vi "banda.vi"() -> ()   [LabVIEW 2020]
uses:
  Control 4.ctl
  <vilib>/Utility/miscctls.llb/LVPointTypeDef.ctl
panel:
  in  "Speed":u8=1
  out "Indicadores":T1
  in  "Start":bool
  in  "Slide":u8(slide) scale=0.0..100.0
  out "Sensores":T2
  # "41-59"
  # "ON"
  # "OFF"
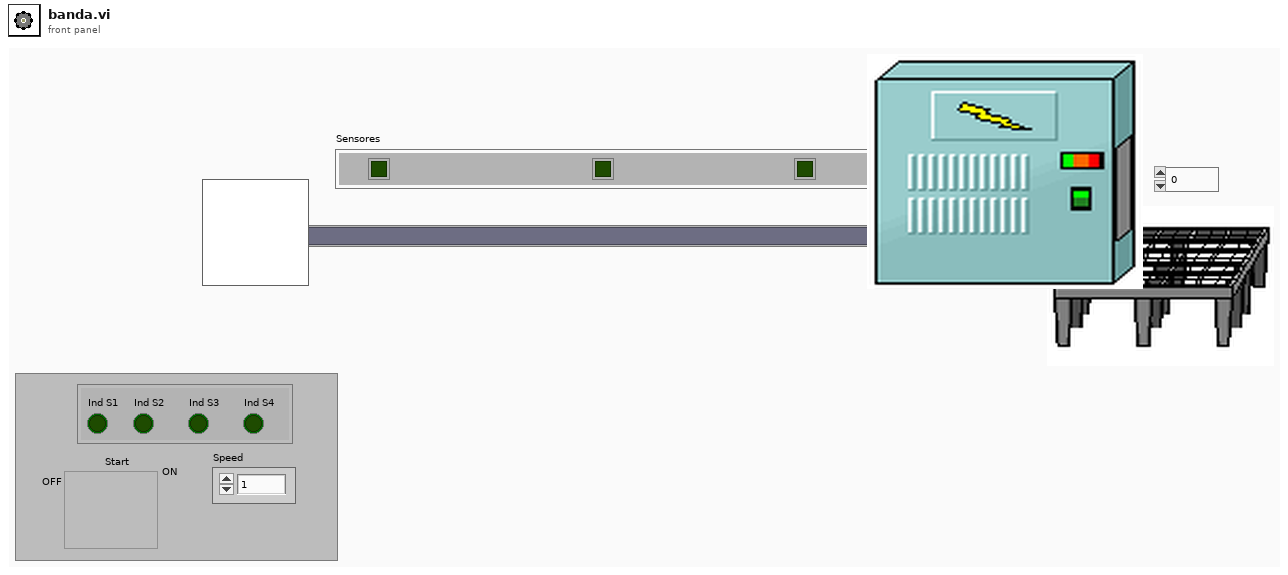
[diagram p1: front panel]
types:
  T1 = cluster{"Ind S1":bool, "Ind S2":bool, "Ind S3":bool, "Ind S4":bool}
  T2 = cluster{"S1":bool, "S2":bool, "S3":bool, "S4":bool}
  T3 = typedef "LVPointTypeDef.ctl" = cluster{"Horizontal":i16, "Vertical":i16}
  T4 = typedef "Control 4.ctl" = enum16{"inicializar", "avanzar", "parar", "verificar"}
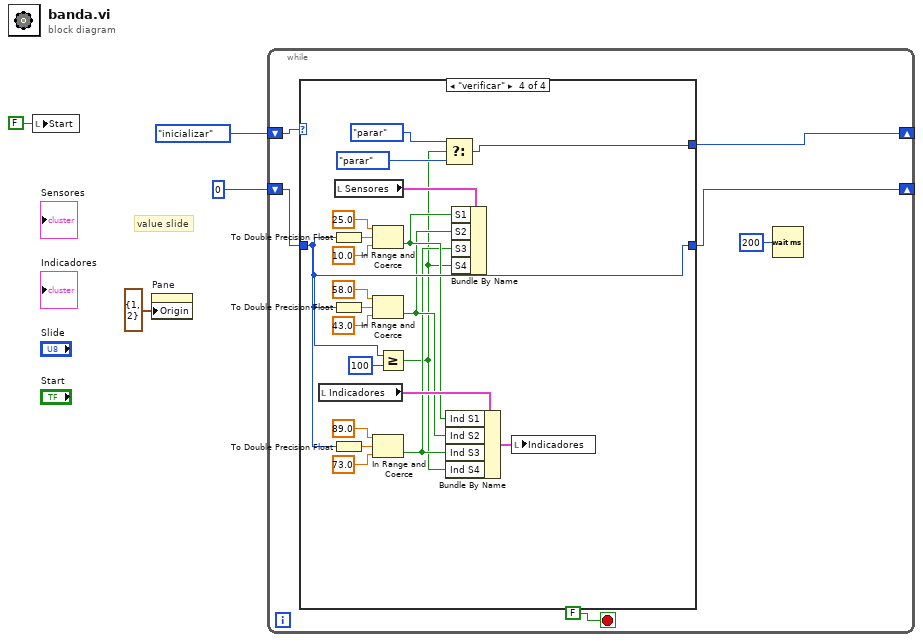
[diagram p0: block diagram]
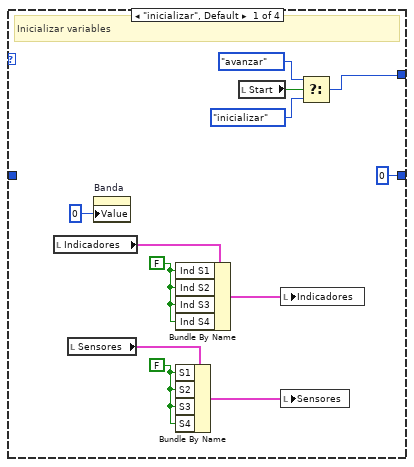
[diagram p2: hidden frame]
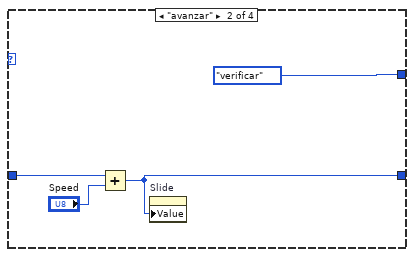
[diagram p3: hidden frame]
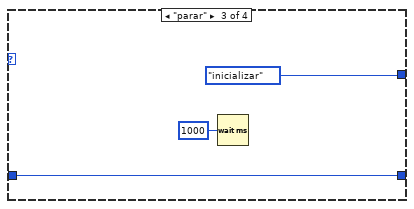
[diagram p4: hidden frame]
diagram:
  # "value slide"
  n1 = local write "Start"(FALSE ("Start")) -> ()
  n2 = property on="Pane" class="Pane"("Origin"=T3 {"Horizontal"=1, "Vertical"=2}) -> ()  [unwired: 2 in, 2 out]
  n3 = while {
    shift-right: [w9] -> _
    shift-left: Control_4."inicializar" -> [w10]
    shift-right: [w7] -> _
    shift-left: u8 0 -> [w8]
    stop <- FALSE stop-if-true
    n4 = case shown="\"verificar\"" w10 {
      tunnel: [w12 Control_4."verificar" Control_4."inicializar" w36] -> w9
      tunnel: w8 -> [_ w26 w29 w39]
      tunnel: [u8 0 w24 w29 w39] -> w7
      frame "inicializar", Default {
        w17 = FALSE ("S1")
        w20 = FALSE ("S1")
        # "Inicializar variables"
        n5 = local read "Indicadores"() -> (w16:T1)
        n6 = local read "Sensores"() -> (w21:T2)
        n7 = property on="Banda" class="Slide (strict)"("Value"=u8 0 ("Slide")) -> ()  [unwired: 2 in, 2 out]
        n8 = Bundle By Name(cluster=w16, "Ind S1"=w17, "Ind S2"=w17, "Ind S3"=w17, "Ind S4"=w17) -> (w18:T1)
        n9 = Bundle By Name(cluster=w21, "S1"=w20, "S2"=w20, "S3"=w20, "S4"=w20) -> (w19:T2)
        n10 = local read "Start"() -> (w15:bool)
        n11 = local write "Indicadores"(w18) -> ()
        n12 = local write "Sensores"(w19) -> ()
        n13 = Select(t=Control_4."avanzar", s=w15, f=Control_4."inicializar") -> (s? t:f=w12:T4)
      }
      frame "avanzar" {
        n14 = Add(x=w26, y="Speed") -> (x+y=w24:u8)
        n15 = property on="Slide" class="Slide (strict)"("Value"=w24) -> ()  [unwired: 2 in, 2 out]
      }
      frame "parar" {
        n16 = Wait (ms)(milliseconds to wait=u32 1000) -> ()  [unwired: 1 out]
      }
      frame "verificar" {
        n17 = local read "Indicadores"() -> (w34:T1)
        n18 = To Double Precision Float(number=w39) -> (double precision float=w48:dbl)
        n19 = To Double Precision Float(number=w39) -> (double precision float=w46:dbl)
        n20 = To Double Precision Float(number=w39) -> (double precision float=w41:dbl)
        n21 = local read "Sensores"() -> (w47:T2)
        n22 = In Range and Coerce(upper limit=25.0 ("lower limit"), x=w48, lower limit=10.0) -> (In Range?=w33:bool)  [unwired: 1 out]
        n23 = In Range and Coerce(upper limit=58.0 ("lower limit"), x=w46, lower limit=43.0) -> (In Range?=w32:bool)  [unwired: 1 out]
        n24 = In Range and Coerce(upper limit=89.0 ("lower limit"), x=w41, lower limit=73.0) -> (In Range?=w31:bool)  [unwired: 1 out]
        n25 = Greater Or Equal?(x=w39, y=u8 100 ("lower limit")) -> (x >= y?=w30:bool)
        n26 = Select(t=Control_4."parar", s=w30, f=Control_4."parar") -> (s? t:f=w36:T4)
        n27 = Bundle By Name(cluster=w34, "Ind S1"=w33, "Ind S2"=w32, "Ind S3"=w31, "Ind S4"=w30) -> (w35:T1)
        n28 = Bundle By Name(cluster=w47, "S1"=w33, "S2"=w32, "S3"=w31, "S4"=w30) -> ()  [unwired: 1 out]
        n29 = local write "Indicadores"(w35) -> ()
      }
    }
    n30 = Wait (ms)(milliseconds to wait=u32 200) -> ()  [unwired: 1 out]
  }
